vi "GetAndFormatDateAndTime.vi"() -> (1 "Date&Time":string)   [LabVIEW 2018]
doc: "Returns a nicely formatted date time string, suitable for use as part of a filename or data log output.\n\nDefault format is:\n\n<Month>_<Day>_<Year>-<Hour>_<Minute>_<Second>\n\nsuch as:\n03_20_2010-13_07_35\n\nCopyright © 2019 Epimedia, Inc. All Rights Reserved.\n\nThe Epimedia Application Library is Copyright © 2009-2017 Epimedia, Inc. \nAll Rights Reserved. Used under license."
panel:
  # "Copyright © 2019 Epimedia, Inc. All Rights Reserved.\n\nThe Epimedia Application Library is Copyright © 2009-2017 Epimedia, Inc. \nAll Rights Reserved. Used under license."
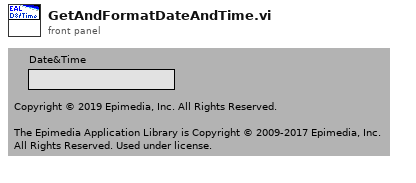
[diagram p1: front panel]
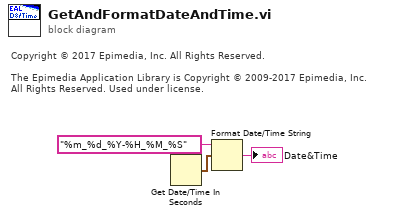
[diagram p0: block diagram]
diagram:
  # "Copyright © 2017 Epimedia, Inc. All Rights Reserved.\n\nThe Epimedia Application Library is Copyright © 2009-2017 Epimedia, Inc. \nAll Rights Reserved. Used under license."
  n1 = Get Date/Time In Seconds() -> (seconds since 1Jan1904=w3:timestamp)
  n2 = Format Date/Time String(time format string (%c)="%m_%d_%Y-%H_%M_%S", seconds (now)=w3) -> (date/time string=→"Date&Time":string)  [unwired: 1 out]
